vi "populateEventSummaryState.vi"(8 "error in (no error)":errorcluster, 11 "Model in":refnum<class "Model.lvclass">) -> (0 "error out":errorcluster, 3 "Model out":refnum<class "Model.lvclass">)   [LabVIEW 2016, in "Model.lvclass"]
uses:
  Model.lvclass
  Model.lvclass/Model.ctl
  Publisher/Publisher.lvclass/Publisher.ctl
  Publisher/Publisher.lvclass
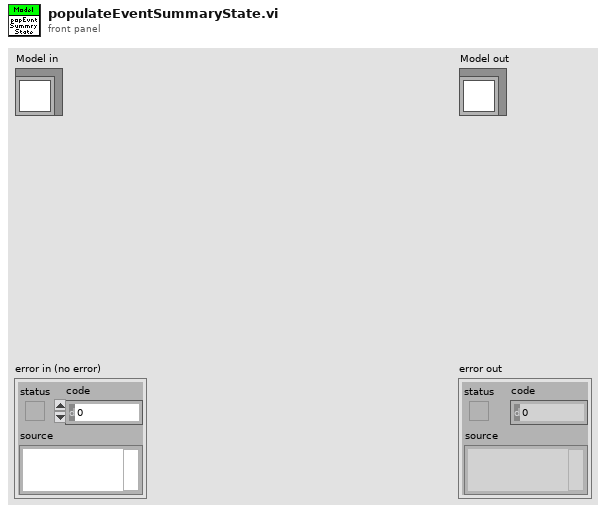
[diagram p1: front panel]
types:
  T1 = typedef "M1M3SupportTopics.lvlib/SummaryStates.ctl" = enum16{"OfflineState", "StandbyState", "DisabledState", "EnabledState", "FaultState"}
  T2 = typedef "M1M3SupportTopics.lvlib/Timestamp.ctl" = dbl
  T3 = typedef "M1M3SupportTopics.lvlib/EventSummaryState.ctl" = cluster{"Timestamp":T2, "SummaryStates":T1}
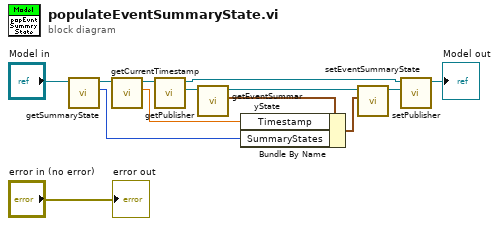
[diagram p0: block diagram]
diagram:
  n1 = call "getSummaryState.vi"("Model in"="Model in") -> ("SummaryStates"=w7:T1, "Model out"=w10:refnum<class "Model.lvclass">)  [unwired: 9 in]
  n2 = call "getCurrentTimestamp.vi"("Model in"=w10) -> ("Timestamp"=w8:T2, "Model out"=w9:refnum<class "Model.lvclass">)  [unwired: 8 in, 1 out]
  n3 = call "getPublisher.vi"("Model in"=w9) -> ("Publisher"=w12:refnum<class "Publisher.lvclass">, "Model out"=w3:refnum<class "Model.lvclass">)  [unwired: 9 in]
  n4 = call "getEventSummaryState.vi"("Publisher in"=w12) -> ("EventSummaryState"=w11:T3, "Publisher out"=w5:refnum<class "Publisher.lvclass">)  [unwired: 9 in]
  n5 = Bundle By Name(cluster=w11, "Timestamp"=w8, "SummaryStates"=w7) -> (w6:T3)
  n6 = call "setEventSummaryState.vi"("EventSummaryState"=w6, "Publisher in"=w5) -> ("Publisher out"=w4:refnum<class "Publisher.lvclass">)  [unwired: 9 in]
  n7 = call "setPublisher.vi"("Publisher"=w4, "Model in"=w3) -> ("Model out"=→"Model out":refnum<class "Model.lvclass">)  [unwired: 9 in]
  "error out" <- "error in (no error)"
